vi "FIFO Test Backup.vi"() -> ()   [LabVIEW 2013]
uses:
  Chroma_ARC_v0.72E/Chroma_ARC_v0.72E/FPGA_Conveyor/5 Channel Timer FGV for FPGA.ctl
  <vilib>/rvi/Emulation/niFpgaSctlEmulationGetInTimedLoop.vi
  <vilib>/rvi/Emulation/niFpgaEmulationReportErrorSimple.vi
  <vilib>/rvi/Emulation/niFpgaGetClockAttributes.vi
  <vilib>/rvi/interface/RandomDataEmulation/nirviRandomDataFPGAFIFO.vi
  <vilib>/rvi/interface/RandomDataEmulation/niFpgaRandomDataHandleErrors.vi
  <vilib>/rvi/Emulation/niFpgaCriticalErrorInLSC.vi
  <vilib>/rvi/DataTransferAndStorage/Container/XNode/niFpgaContainer.xnode
  <vilib>/rvi/interface/RandomDataEmulation/nirviRandomDataFpgaReadWriteTemplate.vi
panel:
  out "T. FIFO Write Timed Out?":bool
  in  "Timer Index":i32
  in  "Timer Target (ticks)":u32
  in  "Set Timer":bool
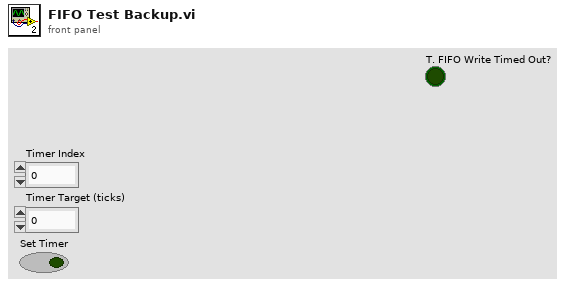
[diagram p1: front panel]
types:
  T1 = typedef "5 Channel Timer FGV for FPGA.ctl" = enum16{"Init Timer", "Set Timer", "Read Time"}
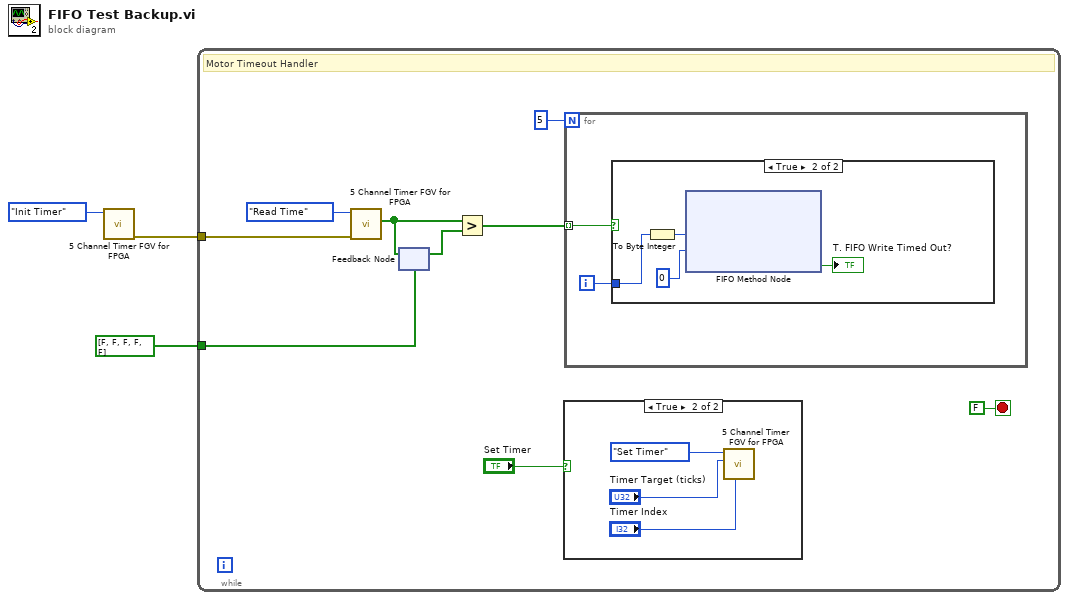
[diagram p0: block diagram]
diagram:
  n1 = call "5 Channel Timer FGV for FPGA.vi"("Timer Mode"=5_Channel_Timer_FGV_for_FPGA."Init Timer") -> ("Error Out"=w2:errorcluster)  [unwired: 7 in, 3 out]
  n2 = while {
    tunnel: w2 -> [w7]
    tunnel: bool[] [FALSE, FALSE, FALSE, FALSE, FALSE] -> [w5]
    stop <- FALSE stop-if-true
    # "Motor Timeout Handler"
    n3 = call "5 Channel Timer FGV for FPGA.vi"("Error In"=w7, "Timer Mode"=5_Channel_Timer_FGV_for_FPGA."Read Time") -> ("Time Elasped (array)"=w10:bool[])  [unwired: 6 in, 3 out]
    n4 = feedback-in #1(w10) -> ()
    n5 = feedback #1(w5) -> (w9:bool[])
    n6 = Greater?(x=w10, y=w9) -> (0:w8:bool[])
    n7 = case shown="True" "Set Timer" {
      frame False {
      }
      frame True {
        n8 = call "5 Channel Timer FGV for FPGA.vi"("index"="Timer Index", "Time Target (s)"="Timer Target (ticks)", "Timer Mode"=5_Channel_Timer_FGV_for_FPGA."Set Timer") -> ()  [unwired: 5 in, 4 out]
      }
    }
    n9 = for {
      N: 5 -> [_]
      tunnel: w8 -> [w17] mode=indexing
      i -> [w16]
      n10 = case shown="True" w17 {
        tunnel: w16 -> [_ w20]
        frame False {
        }
        frame True {
          n11 = To Byte Integer(number=w20) -> (8bit integer=w19:i8)
          n12 = xnode ("FIFO Method Node")("Element"=w19, "Timeout"=0) -> ("Timed Out?"=→"T. FIFO Write Timed Out?":bool)  [unwired: 1 in, 1 out]
        }
      }
    }
  }
